vi "process.vi"(8 "error in":errorcluster, 9 "result allocation":T1, 10 "parameters":T1, 11 "WaveformAcq runtime in":refnum<class "WaveformAcq runtime.lvclass">) -> (0 "error out":errorcluster, 1 "results":T1, 2 "parameter allocation":T1, 3 "WaveformAcq runtime out":refnum<class "WaveformAcq runtime.lvclass">)   [LabVIEW 2017, in "WaveformAcq runtime.lvclass"]
doc: "Provides an interface for information processing by a module at runtime. While this interface performs no operations, a child should provide an override which may process data in any manner necessary."
uses:
  WaveformAcq runtime.lvclass
  <vilib>/NI/Tag Bus/table/data table.ctl
  WaveformAcq runtime.lvclass/WaveformAcq runtime.ctl
  <vilib>/NI/PowerElectronicsControl/WaveformAcq/RT/ErrorSelector.ctl
  <vilib>/NI/PowerElectronicsControl/WaveformAcq/RT/ReadInterleaved.vi
  <vilib>/NI/PowerElectronicsControl/WaveformAcq/RT/WaveformTask.lvclass
  <vilib>/NI/Tag Bus/table/data table.lvlib
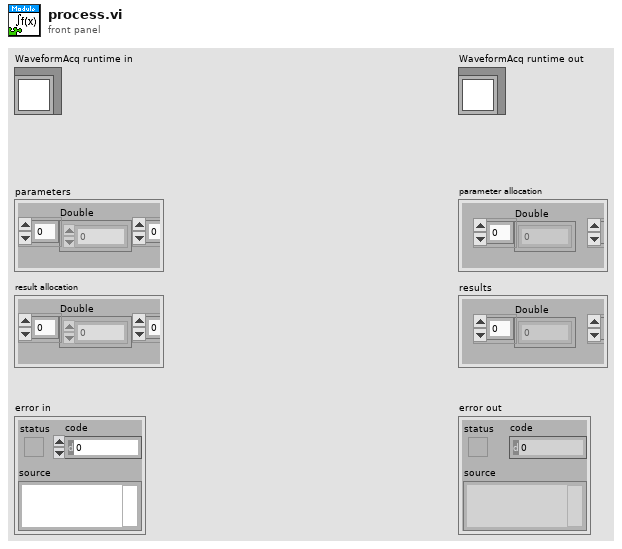
[diagram p1: front panel]
types:
  T1 = typedef "tag bus.lvlib/data table.lvlib/data table.ctl" = cluster{"Double":dbl[], "Single":sgl[], "I64":i64[], "I32":i32[], "I16":i16[], "I8":i8[], "U64":u64[], "U32":u32[], "U16":u16[], "U8":u8[], "Boolean":bool[], "String":string[], "Array of Double":cluster{"DBL Array":dbl[]}[], "Array of Single":cluster{"SGL Array":sgl[]}[], "Array of I64":cluster{"I64 Array":i64[]}[], "Array of I32":cluster{"I32 Array":i32[]}[], "Array of I16":cluster{"I16 Array":i16[]}[], "Array of I8":cluster{"I8 Array":i8[]}[], "Array of U64":cluster{"U64 Array":u64[]}[], "Array of U32":cluster{"U32 Array":u32[]}[], "Array of U16":cluster{"U16 Array":u16[]}[], "Array of U8":cluster{"U8 Array":u8[]}[], "Array of Boolean":cluster{"Boolean Array":bool[]}[], "Array of String":cluster{"String Array":string[]}[]}
  T2 = typedef "WaveformTask.lvclass/ErrorSelector.ctl" = enum16{"Read Timeout", "Module Underflow", "DMA Overflow", "Chan Count", "Run Timeout", "Start Timeout", "Stop Timeout"}
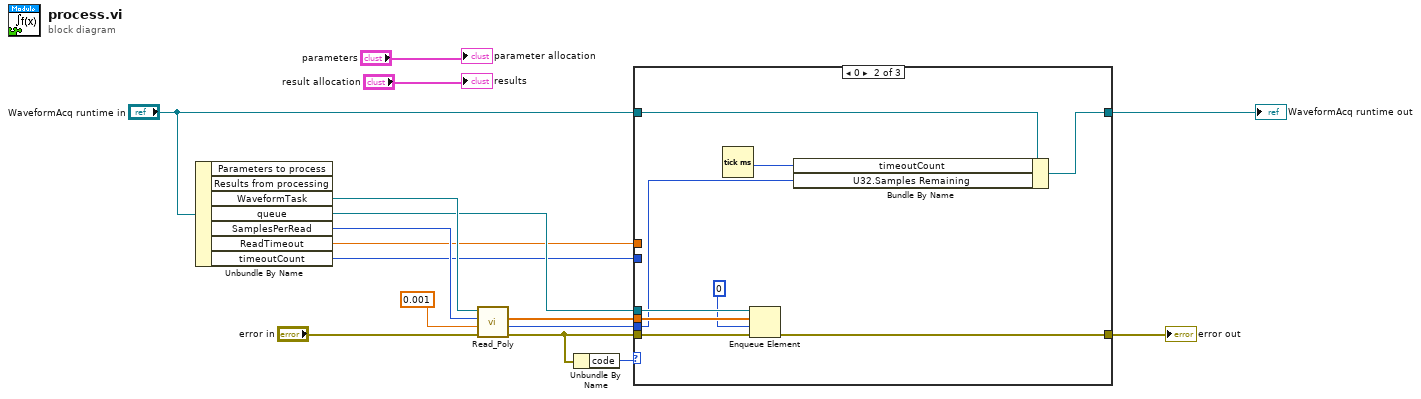
[diagram p0: block diagram]
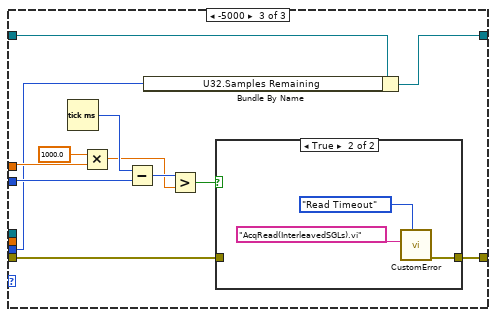
[diagram p3: hidden frame]
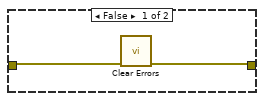
[diagram p4: hidden frame]
diagram:
  n1 = Unbundle By Name("WaveformAcq runtime in") -> ("WaveformTask"=w15:refnum<class "WaveformTask.lvclass">, "queue"=w11:refnum<queue>, "SamplesPerRead"=w14:u32, "ReadTimeout"=w7:dbl, "timeoutCount"=w6:i32)  [unwired: 2 out]
  n2 = call-poly <vilib>:"Read_Poly.vi"("error in"="error in", "Timeout (s)"=0.001, "Samps Read per Chan"=w14, "Task in"=w15) -> ("error out"=w9:errorcluster, "Samples Remaining"=w1:u32, "Data"=w10:sgl[])  [unwired: 4 in, 1 out]
  n3 = Unbundle By Name(w9) -> ("code"=w8:i32)
  n4 = case shown="0" w8 {
    tunnel: w9 -> [w18 w27 w32]
    tunnel: [w18 w26 w31] -> w12
    tunnel: w11 -> [_ w25 _]
    tunnel: w10 -> [_ w24 _]
    tunnel: w7 -> [_ _ w37]
    tunnel: w6 -> [_ _ w39]
    tunnel: "WaveformAcq runtime in" -> [w17 w21 w30]
    tunnel: [w17 w20 w29] -> w4
    tunnel: w1 -> [_ w19 w28]
    frame Default {
    }
    frame 0 {
      n5 = Tick Count (ms)() -> (millisecond timer value=w22:u32)
      n6 = Enqueue Element(queue=w25, element=w24, timeout in ms (-1)=0, error in (no error)=w27) -> (error out=w26:errorcluster)  [unwired: 2 out]
      n7 = Bundle By Name(cluster=w21, "timeoutCount"=w22, "U32.Samples Remaining"=w19) -> (w20:refnum<class "WaveformAcq runtime.lvclass">)
    }
    frame -5000 {
      n8 = Tick Count (ms)() -> (millisecond timer value=w38:u32)
      n9 = Multiply(x=1000.0, y=w37) -> (x*y=w34:dbl)
      n10 = Subtract(x=w38, y=w39) -> (x-y=w35:u32)
      n11 = Bundle By Name(cluster=w30, "U32.Samples Remaining"=w28) -> (w29:refnum<class "WaveformAcq runtime.lvclass">)
      n12 = Greater?(x=w35, y=w34) -> (0:w33:bool)
      n13 = case shown="True" w33 {
        tunnel: w32 -> [w41 _]
        tunnel: [w40 w42] -> w31
        frame False {
          n14 = call <vilib>:"Clear Errors.vi"("error in (no error)"=w41) -> ("error out"=w40:errorcluster)  [unwired: 5 in, 1 out]
        }
        frame True {
          n15 = call <vilib>:"CustomError.vi"("Error Selector"=ErrorSelector."Read Timeout", "VI name"="AcqRead(InterleavedSGLs).vi" ("Calling VI")) -> ("error out"=w42:errorcluster)  [unwired: 9 in]
        }
      }
    }
  }
  "error out" <- w12
  "WaveformAcq runtime out" <- w4
  "results" <- "result allocation"
  "parameter allocation" <- "parameters"
